vi "Read Teller.vi"(11 "Msg Input in":refnum<class "Msg Input.lvclass">) -> (2 "Teller":refnum<class "Teller.lvclass">)   [LabVIEW 2020, in "jettl.lvlib" / "Msg Input.lvclass"]
uses:
  Msg Input.lvclass
  Teller/Teller.lvclass
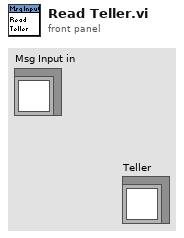
[diagram p1: front panel]
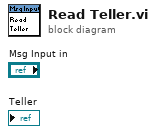
[diagram p0: block diagram]
diagram:
